vi "System-ExecInfo.vi"(1 "Loop Period [ms]":u32, 2 "DSI Reference":refnum<class "DCM-DSI.lvclass">) -> ()   [LabVIEW 2016, in "DSI-RT.lvlib"]
uses:
  DSI-RT.lvlib
  Classes/DCM-DSI/DCM-DSI.lvclass
  <vilib>/Powertrain Controls/Device Drivers/DCM/Rev0/RT/DCM - RT.lvclass/DCM - RT.ctl
  <vilib>/Powertrain Controls/Device Drivers/DCM/Rev0/RT/Read System.vi
  Classes/DCM-DSI/Read DCM Ref.vi
  <vilib>/addons/Software Calibration Management/xSCM/CalPoint.xnode
  <vilib>/Powertrain Controls/Device Drivers/DCM/Rev0/RT/DCM - RT.lvclass
  <vilib>/NI_Real-Time Target Support.lvlib
  <resource>/objmgr/nisysapi.rc
  <vilib>/addons/Software Calibration Management/xSCM/ni_scm.dll
  <vilib>/nisyscfg/nisyscfg.lvlib
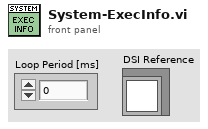
[diagram p1: front panel]
types:
  T1 = typedef "DCM - RT.lvclass/System.ctl" = cluster{"Model":u16, "Rev Major":u8, "Rev Minor":u8, "Serial Number":u32}
  T2 = typedef "NI_Real-Time Target Support.lvlib/RT CPU Load.ctl" = cluster{"Total (%)":dbl, "Time Critical (%)":dbl, "Timed Structures (%)":dbl, "High (%)":dbl, "Above Normal (%)":dbl, "Normal (%)":dbl, "Background (%)":dbl, "Idle (%)":dbl, "ISR (%)":dbl}
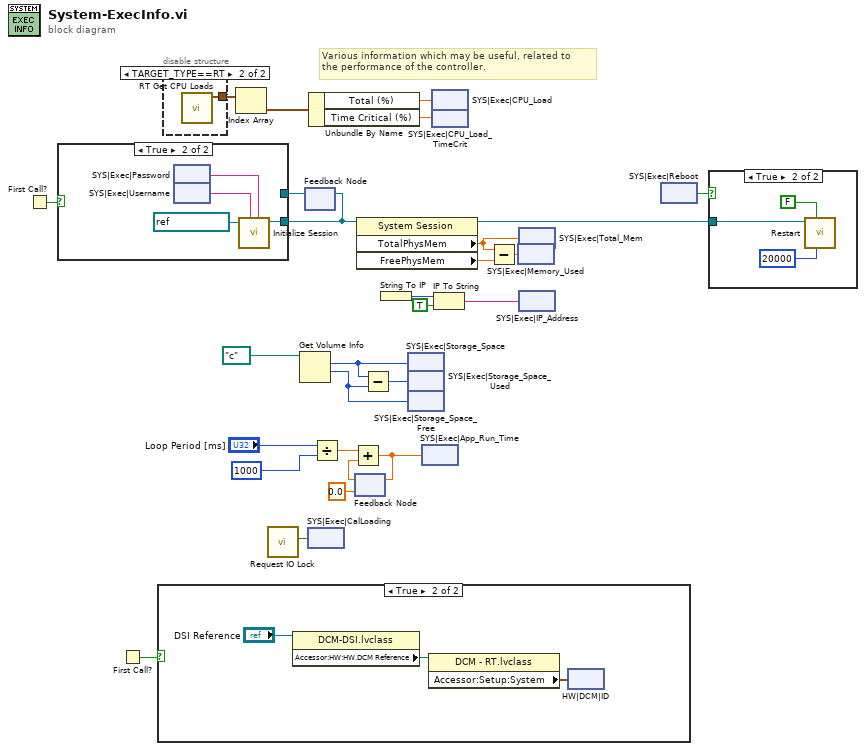
[diagram p0: block diagram]
diagram:
  # "Various information which may be useful, related to\nthe performance of the controller."
  n1 = First Call?() -> (First Call?: T/F=w7:bool)
  n2 = First Call?() -> (First Call?: T/F=w10:bool)
  n3 = case shown="True" w10 {
    frame False {
    }
    frame True {
      n4 = property class="DCM-DSI.lvclass"(reference="DSI Reference") -> ("Accessor:HW:HW.DCM Reference"=w29:refnum<class "DCM - RT.lvclass">)  [unwired: 1 in, 2 out]
      n5 = property class="DCM - RT.lvclass"(reference=w29) -> ("Accessor:Setup:System"=w30:T1)  [unwired: 1 in, 2 out]
      n6 = xnode "HW|DCM|ID"("Value"=w30) -> ()
    }
  }
  n7 = disable-structure shown="TARGET_TYPE==RT" {
    disable-tunnel: [_ w36] -> w18
    frame condition #0 {
    }
    frame condition #1 (active) {
      n8 = call <vilib>:"RT Get CPU Loads.vi"() -> ("CPU loads"=w36:T2[])  [unwired: 10 in, 1 out]
    }
  }
  n9 = Index Array(array=w18) -> (element=w19:T2)  [unwired: 1 in]
  n10 = call <vilib>:"Request IO Lock.vi"() -> ("Request I/O Lock"=w1:bool)  [unwired: 11 in]
  n11 = Get Volume Info(11:path "c:/" ("path")) -> (1:w27:i64, 2:w25:i64)  [unwired: 1 in, 4 out]
  n12 = feedback #1() -> (w5:refnum<k21>)  [unwired: 1 in]
  n13 = case shown="True" w7 {
    tunnel: [w37 w41] -> w6
    tunnel: w5 -> [w37 _]
    frame False {
    }
    frame True {
      n14 = xnode "SYS|Exec|Password"() -> ("Value"=w39:string)
      n15 = xnode "SYS|Exec|Username"() -> ("Value"=w40:string)
      n16 = call <vilib>:"Initialize Session.vi"("Password"=w39, "User Name"=w40, "Target (localhost)"=refnum<k21> "localhost") -> ("Session out"=w41:refnum<k21>)  [unwired: 7 in, 1 out]
    }
  }
  n17 = feedback-in #1(w6) -> ()
  n18 = xnode "SYS|Exec|CalLoading"("Value"=w1) -> ()
  n19 = Unbundle By Name(w19) -> ("Total (%)"=w20:dbl, "Time Critical (%)"=w21:dbl)
  n20 = Divide(x="Loop Period [ms]", y=u32 1000) -> (x/y=w12:dbl)
  n21 = feedback #2(0.0) -> (w14:dbl)
  n22 = Add(x=w12, y=w14) -> (x+y=w11:dbl)
  n23 = feedback-in #2(w11) -> ()
  n24 = property class="System Session"(reference=w6) -> (reference out=w8:refnum<k21>, "TotalPhysMem"=w22:dbl, "FreePhysMem"=w23:dbl)  [unwired: 1 in, 1 out]
  n25 = Subtract(x=w25, y=w27) -> (x-y=w26:i64)
  n26 = String To IP() -> (0:w4:u32)  [unwired: 1 in]
  n27 = xnode "SYS|Exec|Storage_Space"("Value"=w25) -> ()
  n28 = xnode "SYS|Exec|Storage_Space_Used"("Value"=w26) -> ()
  n29 = xnode "SYS|Exec|Storage_Space_Free"("Value"=w27) -> ()
  n30 = xnode "SYS|Exec|App_Run_Time"("Value"=w11) -> ()
  n31 = xnode "SYS|Exec|CPU_Load"("Value"=w20) -> ()
  n32 = xnode "SYS|Exec|CPU_Load_TimeCrit"("Value"=w21) -> ()
  n33 = IP To String(1:TRUE ("dot notation? (F)"), 2:w4) -> (0:w2:string)
  n34 = Subtract(x=w22, y=w23) -> (x-y=w17:dbl)
  n35 = xnode "SYS|Exec|Memory_Used"("Value"=w17) -> ()
  n36 = xnode "SYS|Exec|Total_Mem"("Value"=w22) -> ()
  n37 = xnode "SYS|Exec|IP_Address"("Value"=w2) -> ()
  n38 = xnode "SYS|Exec|Reboot"() -> ("Value"=w9:bool)
  n39 = case shown="True" w9 {
    tunnel: w8 -> [_ w69]
    frame False {
    }
    frame True {
      n40 = call <vilib>:"Restart.vi"("Timeout (180,000 ms)"=u32 20000, "Wait Until Complete (T)"=FALSE, "Session in"=w69) -> ()  [unwired: 6 in, 3 out]
    }
  }
